vi "Read Data2D.lvclass.vi"(8 "error in (no error)":errorcluster, 11 "IV in":refnum<class "IV.lvclass">) -> (0 "error out":errorcluster, 2 "Data2D.lvclass":refnum<class "Data2D.lvclass">, 3 "IV out":refnum<class "IV.lvclass">)   [LabVIEW 2018, in "IV.lvclass"]
uses:
  IV.lvclass
  Data/Data2D/Data2D.lvclass
  Experiment/Experiment2D/Experiment2D.lvclass
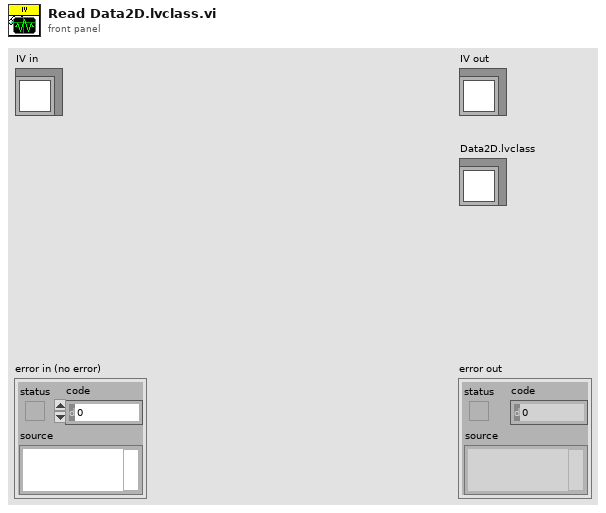
[diagram p1: front panel]
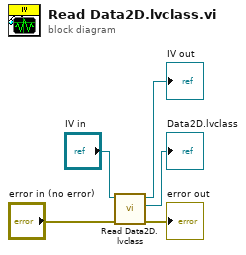
[diagram p0: block diagram]
diagram:
  n1 = call-parent "Read Data2D.lvclass.vi"("error in (no error)"="error in (no error)", "Experiment2D in"="IV in") -> ("error out"=→"error out":errorcluster, "Data2D.lvclass"=→"Data2D.lvclass":refnum<class "Data2D.lvclass">, "Experiment2D out"=→"IV out":refnum<class "IV.lvclass">)  [unwired: 7 in]
